vi "Draw Term Label.vi"(4 "Value Color":u32(colorbox)=32639, 6 "Type Color":u32(colorbox)=32639, 7 "Bounds":T1={"left"=0, "top"=0, "right"=150, "bottom"=100}, 9 "Value":string, 10 "Name":string, 11 "Picture In":picture) -> (3 "Picture":picture)   [LabVIEW 2022 SP3, in "FlexBlocks Support.lvlib"]
uses:
  FlexBlocks Support.lvlib
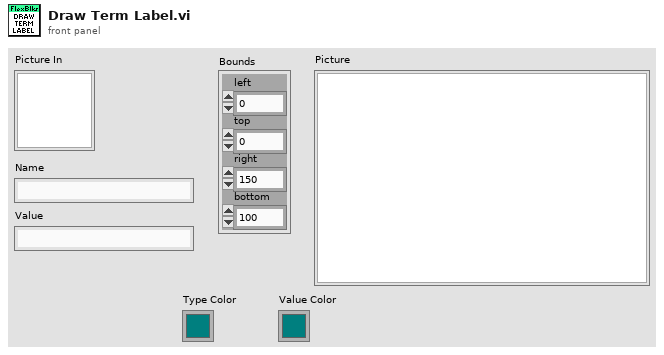
[diagram p1: front panel]
types:
  T1 = cluster{"left":i16, "top":i16, "right":i16, "bottom":i16}
  T2 = typedef "FlexBlocks Support.lvlib/Size Constants.ctl" = cluster{"Icon Size":i32, "Name H Pad":i32, "Name V Pad":i32, "Max Label Width":i32, "Value Width":i32, "Frame Padding":i32, "Vertical Margin":i32, "Min Width":i32, "Min Height":i32, "Collapsed Spacing":i32, "Terminal Center Offset":i32}
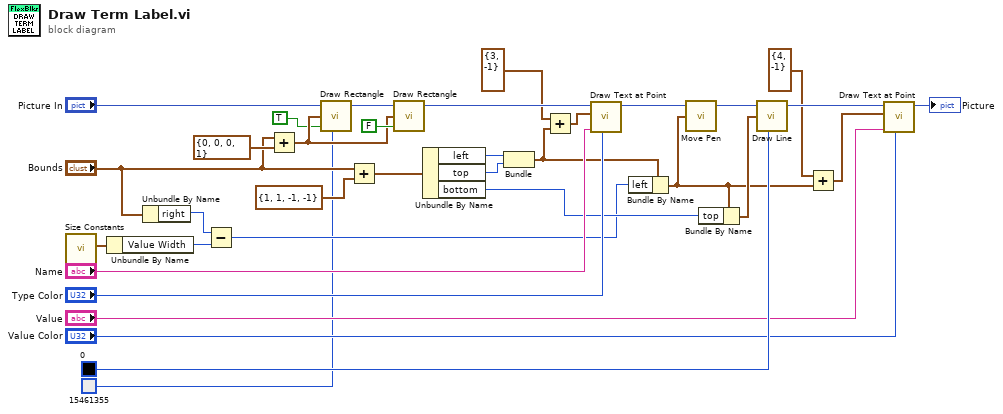
[diagram p0: block diagram]
diagram:
  n1 = call "Size Constants.vi"() -> ("Size Constants"=w9:T2)  [unwired: 11 in]
  n2 = Unbundle By Name(w9) -> ("Value Width"=w8:i32)
  n3 = Unbundle By Name("Bounds") -> ("right"=w7:i16)
  n4 = Subtract(x=w7, y=w8) -> (x-y=w6:i32)
  n5 = Add(x="Bounds", y=T1 {"left"=0, "top"=0, "right"=0, "bottom"=1} ("Frame Border")) -> (x+y=w3:T1)
  n6 = call <vilib>:"Draw Rectangle.vi"("picture"="Picture In", "rect"=w3, "fill?(F)"=TRUE, "color(black)"=u32 15461355) -> ("new picture"=w33:picture)  [unwired: 5 in]
  n7 = Add(x="Bounds", y=T1 {"left"=1, "top"=1, "right"=-1, "bottom"=-1} ("Frame Border")) -> (x+y=w29:T1)
  n8 = call <vilib>:"Draw Rectangle.vi"("picture"=w33, "rect"=w3, "fill?(F)"=FALSE) -> ("new picture"=w30:picture)  [unwired: 6 in]
  n9 = Unbundle By Name(w29) -> ("left"=w28:i16, "top"=w27:i16, "bottom"=w19:i16)
  n10 = Bundle("left"=w28, "top"=w27) -> (w21:cluster{"left":i16, "top":i16})  [unwired: 1 in]
  n11 = Add(x=cluster{"left":i16, "top":i16} {"left"=3, "top"=-1} ("output cluster"), y=w21) -> (x+y=w24:cluster{"left":i16, "top":i16})
  n12 = call <vilib>:"Draw Text at Point.vi"("text color(black)"="Type Color", "text"="Name", "origin"=w24, "picture"=w30) -> ("new picture"=w23:picture)  [unwired: 6 in, 1 out]
  n13 = Bundle By Name(cluster=w21, "left"=w6) -> (w16:cluster{"left":i16, "top":i16})
  n14 = call <vilib>:"Move Pen.vi"("new position"=w16, "picture"=w23) -> ("new picture"=w22:picture)  [unwired: 3 in]
  n15 = Bundle By Name(cluster=w16, "top"=w19) -> (w18:cluster{"left":i16, "top":i16})
  n16 = call <vilib>:"Draw Line.vi"("picture"=w22, "end point"=w18, "color(black)"=u32 0) -> ("new picture"=w17:picture)  [unwired: 6 in]
  n17 = Add(x=cluster{"left":i16, "top":i16} {"left"=4, "top"=-1} ("output cluster"), y=w16) -> (x+y=w14:cluster{"left":i16, "top":i16})
  n18 = call <vilib>:"Draw Text at Point.vi"("text color(black)"="Value Color", "text"="Value", "origin"=w14, "picture"=w17) -> ("new picture"=→"Picture":picture)  [unwired: 6 in, 1 out]
